vi "SeCrTS-DD signal names extracter.vi"(11 "input cluster":T1) -> (3 "Signal names":T2)   [LabVIEW 2022 SP3]
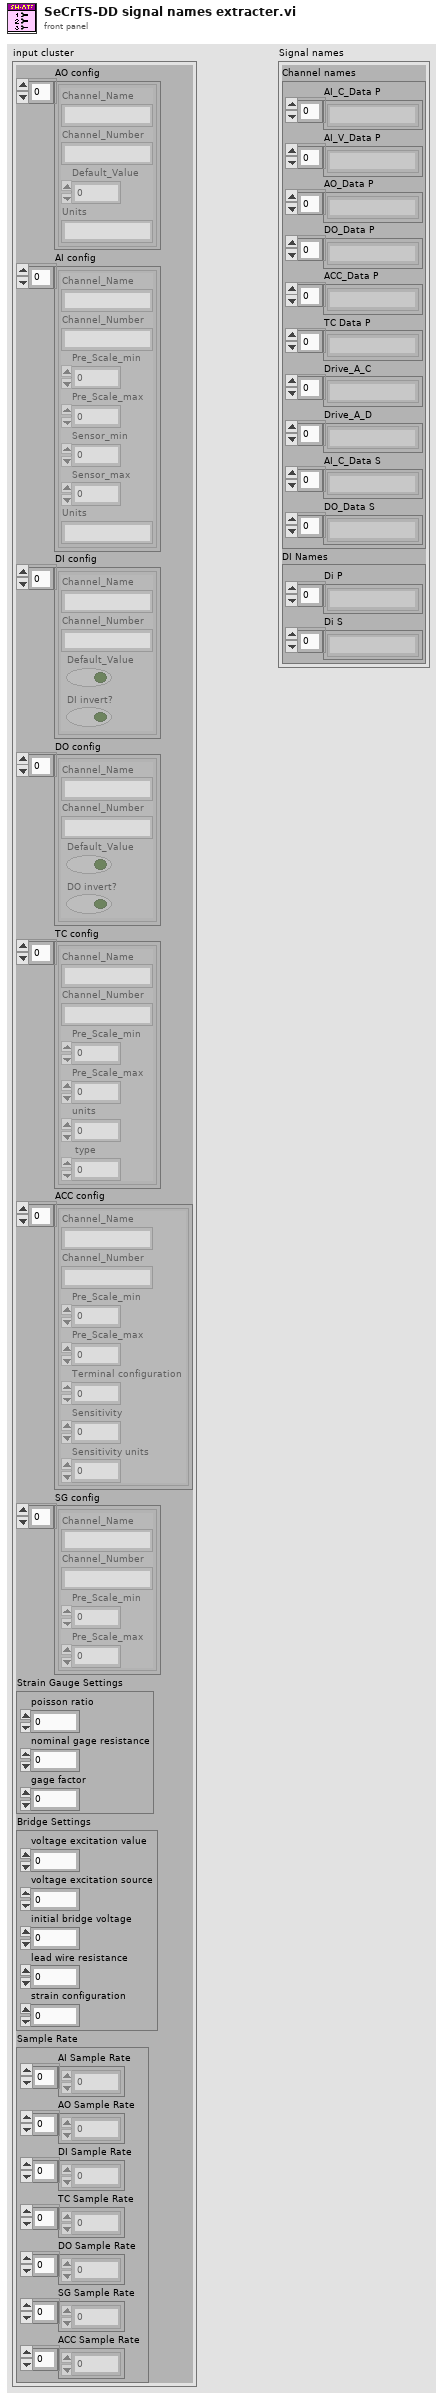
[diagram p1: front panel]
types:
  T1 = cluster{"AO config":cluster{"Channel_Name":string, "Channel_Number":string, "Default_Value":dbl, "Units":string}[], "AI config":cluster{"Channel_Name":string, "Channel_Number":string, "Pre_Scale_min":dbl, "Pre_Scale_max":dbl, "Sensor_min":dbl, "Sensor_max":dbl, "Units":string}[], "DI config":cluster{"Channel_Name":string, "Channel_Number":string, "Default_Value":bool, "DI invert?":bool}[], "DO config":cluster{"Channel_Name":string, "Channel_Number":string, "Default_Value":bool, "DO invert?":bool}[], "TC config":cluster{"Channel_Name":string, "Channel_Number":string, "Pre_Scale_min":dbl, "Pre_Scale_max":dbl, "units":i32, " type":i32}[], "ACC config":cluster{"Channel_Name":string, "Channel_Number":string, "Pre_Scale_min":dbl, "Pre_Scale_max":dbl, "Terminal configuration":i32, "Sensitivity":dbl, "Sensitivity units":i32}[], "SG config":cluster{"Channel_Name":string, "Channel_Number":string, "Pre_Scale_min":dbl, "Pre_Scale_max":dbl}[], "Strain Gauge Settings":cluster{"poisson ratio":dbl, "nominal gage resistance":dbl, "gage factor":dbl}, "Bridge Settings":cluster{"voltage excitation value":dbl, "voltage excitation source":i32, "initial bridge voltage":dbl, "lead wire resistance":dbl, "strain configuration":i32}, "Sample Rate":cluster{"AI Sample Rate":dbl[], "AO Sample Rate":dbl[], "DI Sample Rate":dbl[], "TC Sample Rate":dbl[], "DO Sample Rate":dbl[], "SG Sample Rate":dbl[], "ACC Sample Rate":dbl[]}}
  T2 = cluster{"Channel names":cluster{"AI_C_Data P":string[], "AI_V_Data P":string[], "AO_Data P":string[], "DO_Data P":string[], "ACC_Data P":string[], "TC Data P":string[], "Drive_A_C":string[], "Drive_A_D":string[], "AI_C_Data S":string[], "DO_Data S":string[]}, "DI Names":cluster{"Di P":string[], "Di S":string[]}}
  T3 = cluster{"Channel_Name":string, "Channel_Number":string, "Default_Value":dbl, "Units":string}[]
  T4 = cluster{"Channel_Name":string, "Channel_Number":string, "Pre_Scale_min":dbl, "Pre_Scale_max":dbl, "Sensor_min":dbl, "Sensor_max":dbl, "Units":string}[]
  T5 = cluster{"Channel_Name":string, "Channel_Number":string, "Default_Value":bool, "DI invert?":bool}[]
  T6 = cluster{"Channel_Name":string, "Channel_Number":string, "Default_Value":bool, "DO invert?":bool}[]
  T7 = cluster{"Channel_Name":string, "Channel_Number":string, "Pre_Scale_min":dbl, "Pre_Scale_max":dbl, "units":i32, " type":i32}[]
  T8 = cluster{"Channel_Name":string, "Channel_Number":string, "Pre_Scale_min":dbl, "Pre_Scale_max":dbl, "Terminal configuration":i32, "Sensitivity":dbl, "Sensitivity units":i32}[]
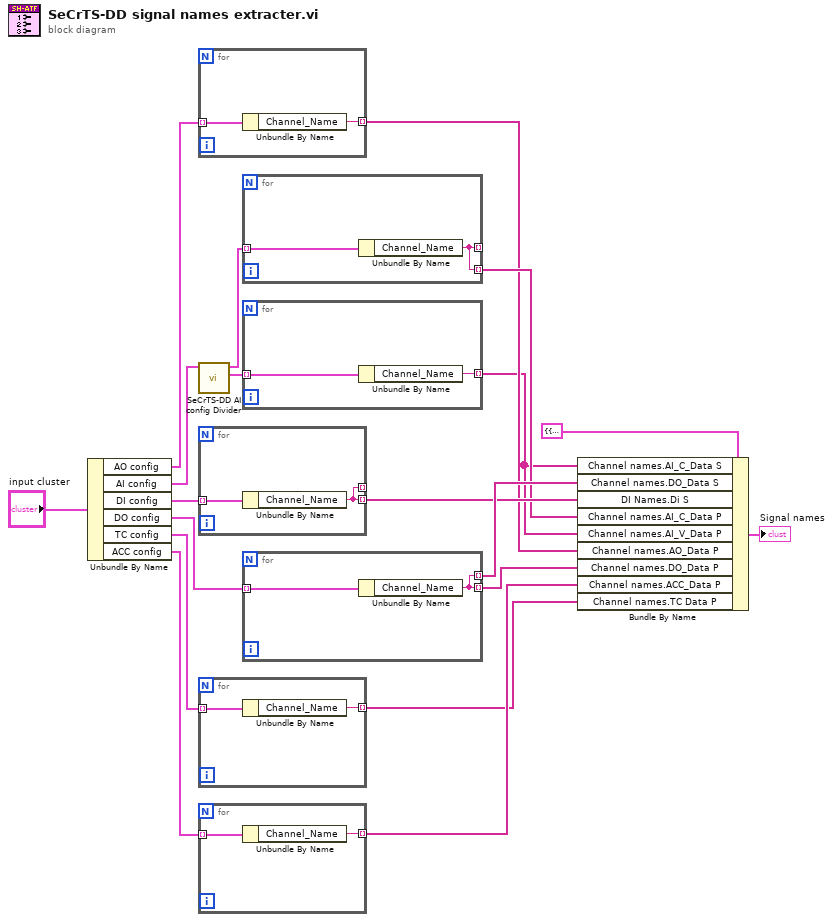
[diagram p0: block diagram]
diagram:
  n1 = Unbundle By Name("input cluster") -> ("AO config"=w12:T3, "AI config"=w17:T4, "DI config"=w13:T5, "DO config"=w14:T6, "TC config"=w15:T7, "ACC config"=w16:T8)
  n2 = for {
    tunnel: w12 -> [w21] mode=indexing
    tunnel: [w20] -> w7 mode=indexing
    n3 = Unbundle By Name(w21) -> ("Channel_Name"=w20:string)
  }
  n4 = call "SeCrTS-DD AI config Divider.vi"("AI config"=w17) -> ("AI V"=w19:T4, "AI C"=w18:T4)  [unwired: 9 in]
  n5 = for {
    tunnel: [w22] -> _ mode=indexing
    tunnel: w13 -> [w23] mode=indexing
    tunnel: [w22] -> w9 mode=indexing
    n6 = Unbundle By Name(w23) -> ("Channel_Name"=w22:string)
  }
  n7 = for {
    tunnel: [w25] -> w4 mode=indexing
    tunnel: w15 -> [w24] mode=indexing
    n8 = Unbundle By Name(w24) -> ("Channel_Name"=w25:string)
  }
  n9 = for {
    tunnel: w16 -> [w27] mode=indexing
    tunnel: [w26] -> w5 mode=indexing
    n10 = Unbundle By Name(w27) -> ("Channel_Name"=w26:string)
  }
  n11 = for {
    tunnel: w18 -> [w29] mode=indexing
    tunnel: [w28] -> w8 mode=indexing
    tunnel: [w28] -> _ mode=indexing
    n12 = Unbundle By Name(w29) -> ("Channel_Name"=w28:string)
  }
  n13 = for {
    tunnel: w19 -> [w31] mode=indexing
    tunnel: [w30] -> w1 mode=indexing
    n14 = Unbundle By Name(w31) -> ("Channel_Name"=w30:string)
  }
  n15 = for {
    tunnel: w14 -> [w33] mode=indexing
    tunnel: [w32] -> w6 mode=indexing
    tunnel: [w32] -> w10 mode=indexing
    n16 = Unbundle By Name(w33) -> ("Channel_Name"=w32:string)
  }
  n17 = Bundle By Name(cluster=T2 {"Channel names"={"AI_C_Data P"=[], "AI_V_Data P"=[], "AO_Data P"=[], "DO_Data P"=[], "ACC_Data P"=[], "TC Data P"=[], "Drive_A_C"=[], "Drive_A_D"=[], "AI_C_Data S"=[], "DO_Data S"=[]}, "DI Names"={"Di P"=[], "Di S"=[]}} ("Signal names"), "Channel names.AI_C_Data S"=w1, "Channel names.DO_Data S"=w10, "DI Names.Di S"=w9, "Channel names.AI_C_Data P"=w8, "Channel names.AI_V_Data P"=w1, "Channel names.AO_Data P"=w7, "Channel names.DO_Data P"=w6, "Channel names.ACC_Data P"=w5, "Channel names.TC Data P"=w4) -> (→"Signal names":T2)
